vi "ex1.vi"() -> ()   [LabVIEW 2022 SP3]
panel:
  out "String":string
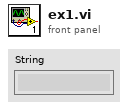
[diagram p1: front panel]
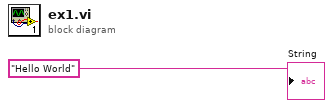
[diagram p0: block diagram]
diagram:
  "String" <- "Hello World"
